vi "File Extension to Delimiter.vi"(8 "error in":errorcluster, 11 "Data File Path":path) -> (0 "error out":errorcluster, 3 "Delimiter":string)   [LabVIEW 2020]
doc: "Outputs the delimiter character (tab or ,), based on the file extension (tsv, csv)."
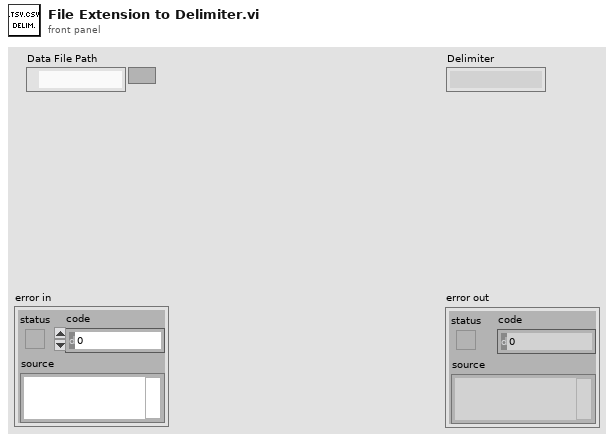
[diagram p1: front panel]
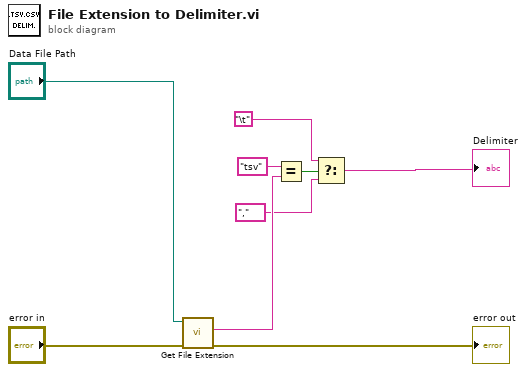
[diagram p0: block diagram]
diagram:
  n1 = call <vilib>:"Get File Extension.vi"("error in (no error)"="error in", "file"="Data File Path") -> ("error out"=→"error out":errorcluster, "lowercase file extension"=w9:string)  [unwired: 5 in, 3 out]
  n2 = Equal?(x="tsv", y=w9) -> (x = y?=w4:bool)
  n3 = Select(t="\t", s=w4, f=",") -> (s? t:f=→"Delimiter":string)
